vi "Room Service Manager.vi"() -> ()   [LabVIEW 2023]
panel:
  in  "Boolean":bool
  in  "Back":bool
  in  "Service State":T1(tab)
  in  "Other Request":bool
  in  "Food Order":bool
  in  "HouseKeeping":bool
  in  "Room Cleaning":bool
  in  "Laundry":bool
  in  "Request":bool
  in  "Request Details":string
  in  "Other Request 2":bool
  # "Room Service: 101"
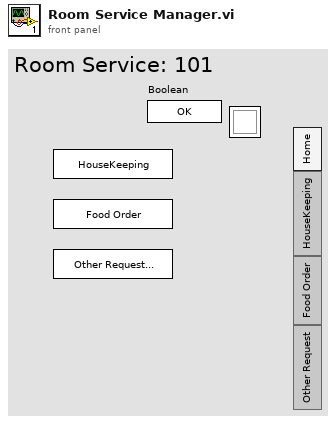
[diagram p1: front panel]
types:
  T1 = enum32{"Home", "HouseKeeping", "Food Order", "Other Request"}
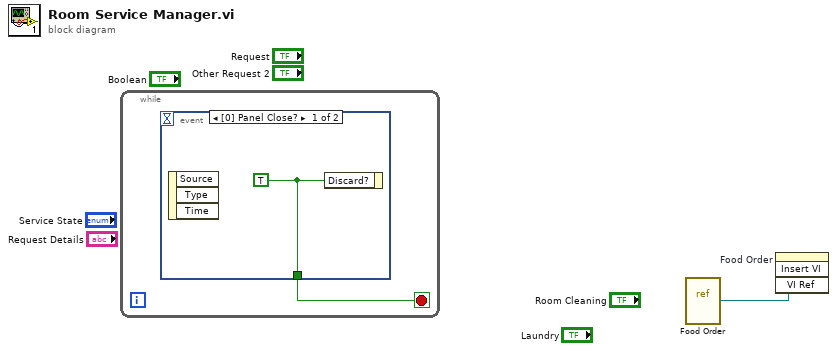
[diagram p0: block diagram]
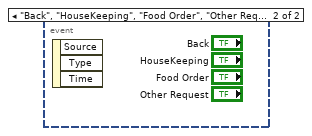
[diagram p2: hidden frame]
diagram:
  n1 = while {
    stop <- w2 stop-if-true
    n2 = event shown="[0] Panel Close?" {
      selector: _ -> [_ _]
      dyn-events: _ -> [_ _]
      timeout: _ -> [_ _]
      tunnel: [w3 _] -> w2
      event Panel Close? {
        w3 = TRUE ("Discard?")
        n3 = event-data() -> ()  [unwired: 1 in, 3 out]
        n4 = event-data("Discard?"=w3) -> ()  [unwired: 1 in, 1 out]
      }
      event "Back", "HouseKeeping", "Food Order", "Other Request": Value Change {
        n5 = event-data() -> ()  [unwired: 1 in, 3 out]
      }
    }
  }
  n6 = vi-ref "Food Order.vi"() -> (w1:refnum<vi>)
  n7 = invoke on="Food Order" class="SubPnl" method="Insert VI"("VI Ref"=w1) -> ()  [unwired: 3 in, 4 out]
